vi "Put Low Extra Temp Alarm V.vi"(8 "error in (no error)":errorcluster, 10 "lowtempExAlarm":sgl, 11 "sensorNumber":i32) -> (0 "error out":errorcluster, 3 "function return":i32)   [LabVIEW 2009, in "VantagePro.lvlib"]
doc: "DllAccess int _stdcall PutLowExtraTempAlarm_V( int sensorNumber, float lowtempExAlarm );"
uses:
  VantagePro.lvlib
  <userlib>/VantagePro/VantagePro.dll
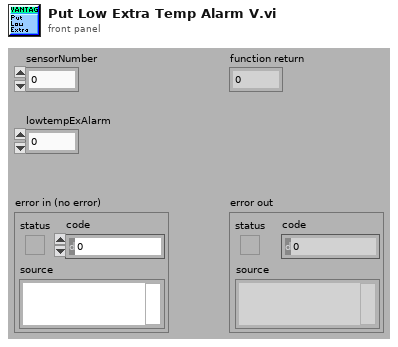
[diagram p1: front panel]
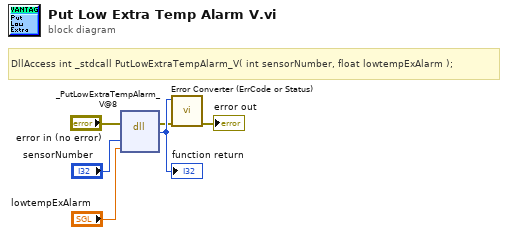
[diagram p0: block diagram]
diagram:
  # "DllAccess int _stdcall PutLowExtraTempAlarm_V( int sensorNumber, float lowtempExAlarm );"
  n1 = dll-call lib="C:/Program Files/National Instruments/LabVIEW 2010/user.lib/VantagePro/VantagePro.*" fn="_PutLowExtraTempAlarm_V@8"(error in="error in (no error)", "sensorNumber"="sensorNumber", "lowtempExAlarm"="lowtempExAlarm") -> (error out=w2:errorcluster, w6:i32)  [unwired: 4 in, 1 out]
  "function return" <- w6
  n2 = call "Error Converter (ErrCode or Status).vi"("error in (no error)"=w2, "error code"=w6) -> ("error out"=→"error out":errorcluster)  [unwired: 9 in]
